vi "FlexDDS-NG_DCP_Channels2String.vi"(11 "Channels":T1(ring)) -> (3 "channels string":string)   [LabVIEW 2016]
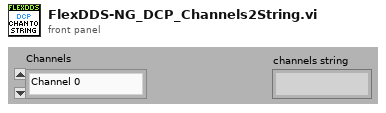
[diagram p1: front panel]
types:
  T1 = enum32{"Channel 0", "Channel 1", "Both channels"}
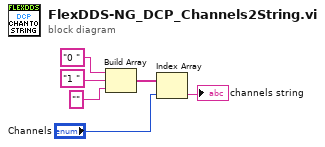
[diagram p0: block diagram]
diagram:
  n1 = Build Array("0 " ("string"), "1 " ("string"), "" ("string")) -> (w3:string[])
  n2 = Index Array(array=w3, index="Channels") -> (element=→"channels string":string)
